vi "Initialize.vi"(5 "Reset (False)":bool, 8 "error in (no error)":errorcluster, 9 "Baud Rate (38400)":u32(ring)=38400 items=["9600"=9600, "19200"=19200, "38400"=38400, "57600"=57600, "115200"=115200, "230400"=230400, "460800"=460800], 10 "Node (3)":u8=3 caption="Node" min=3 max=128 step=1, 11 "VISA resource name":refnum<visa-resource-name>) -> (0 "error out":errorcluster, 3 "VISA resource name out":refnum<visa-resource-name>)   [LabVIEW 2022 SP3, in "Bronkhorst FLOW-BUS.lvlib"]
doc: "Establishes communication with the instrument and needs to be called before calling other instrument driver VIs for this instrument. Generally, you need to call the Initialize VI only once at the beginning of an application."
uses:
  Bronkhorst FLOW-BUS.lvlib
panel:
  # "(c) 2014 Bronkhorst High-Tech B.V.  ALL RIGHTS RESERVED."
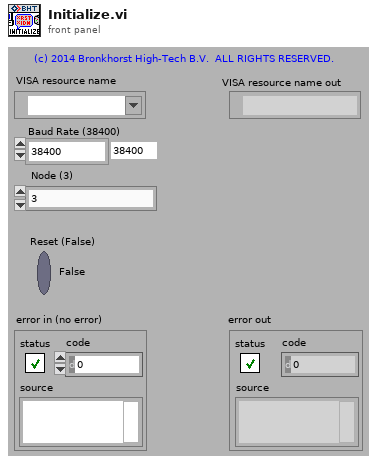
[diagram p1: front panel]
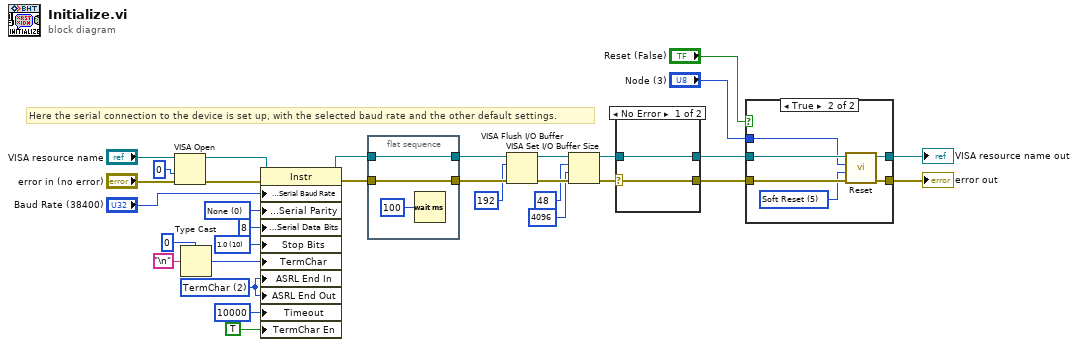
[diagram p0: block diagram]
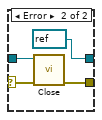
[diagram p3: hidden frame]
diagram:
  w23 = u16 2 items=["None", "Last Bit", "TermChar"] ("Serial Settings:End Mode for Reads")
  w24 = u16 10 items=["1.0"=10, "1.5"=15, "2.0"=20] ("Serial Settings:Stop Bits")
  w26 = u16 0 items=["None", "Odd", "Even", "Mark", "Space"] ("Serial Settings:Parity")
  # "Here the serial connection to the device is set up, with the selected baud rate and the other default settings."
  n1 = VISA Open(access mode=u32 0, error in (no error)="error in (no error)", VISA resource name="VISA resource name") -> (VISA resource name=w22:refnum<visa-resource-name>, error out=w21:errorcluster)  [unwired: 2 in]
  n2 = Type Cast(type=u8 0, x="\n") -> (*(type *) &x=w10:u8)
  n3 = property on="Property Node" class="Instr"(reference=w22, error in=w21, "Serial Settings:Serial Baud Rate"="Baud Rate (38400)", "Serial Settings:Serial Parity"=w26, "Serial Settings:Serial Data Bits"=u16 8 ("Serial Settings:Data Bits"), "Stop Bits"=w24, "TermChar"=w10, "ASRL End In"=w23, "ASRL End Out"=w23, "Timeout"=u32 10000 ("General Settings:Timeout Value"), "TermChar En"=TRUE ("Message Based Settings:Termination Character Enable")) -> (reference out=w29:refnum<visa-resource-name>, error out=w28:errorcluster)
  n4 = flat-sequence {
    tunnel: w29 -> [w35]
    tunnel: w28 -> [w34]
    tunnel: [w35] -> w14
    tunnel: [w34] -> w13
    frame #0 {
      n5 = Wait (ms)(milliseconds to wait=u32 100) -> ()  [unwired: 1 out]
    }
  }
  n6 = VISA Flush I/O Buffer(VISA resource name=w14, mask (16)=u16 192, error in (no error)=w13) -> (VISA resource name out=w20:refnum<visa-resource-name>, error out=w19:errorcluster)
  n7 = VISA Set I/O Buffer Size(VISA resource name=w20, mask (16)=u16 48, size (4096)=u32 4096 ("size (0)"), error in (no error)=w19) -> (VISA resource name out=w8:refnum<visa-resource-name>, error out=w9:errorcluster)
  n8 = case shown="No Error" w9 {
    selector: w9 -> [w36 w39]
    tunnel: w8 -> [w37 w40]
    tunnel: [w37 refnum<visa-resource-name> refnum ("VISA resource name out")] -> w2
    tunnel: [w36 w41] -> w1
    frame No Error {
    }
    frame Error {
      n9 = call "Close.vi"("error in (no error)"=w39, "VISA resource name"=w40) -> ("error out"=w41:errorcluster)  [unwired: 9 in]
    }
  }
  n10 = case shown="True" "Reset (False)" {
    tunnel: w1 -> [w42 w49]
    tunnel: w2 -> [w43 w48]
    tunnel: "Node (3)" -> [_ w45]
    tunnel: [w43 w47] -> w5
    tunnel: [w42 w46] -> w4
    frame False {
    }
    frame True {
      w44 = u32 5 items=["No Reset", "Reset counter value (no mode change)", "Reset alarm", "Restart batch counter", "Reset counter value (counter off)", "Soft Reset"] ("Reset mode (5: Soft Reset)")
      n11 = call "Reset.vi"("error in (no error)"=w49, "Reset mode (5: Soft Reset)"=w44, "Node (3)"=w45, "VISA resource name"=w48) -> ("error out"=w46:errorcluster, "VISA resource name out"=w47:refnum<visa-resource-name>)  [unwired: 6 in]
    }
  }
  "VISA resource name out" <- w5
  "error out" <- w4
